vi "Tx Cyclic Init.vi"(8 "error in (no error)":errorcluster, 9 "Channel Number":u32, 10 "signal list":refnum<k21>[](array[refnum])=["CANCyclicSignal1\nnixnet_example.CAN_Cluster", "CANCyclicSignal2\nnixnet_example.CAN_Cluster", "CANCyclicSignal3\nnixnet_example.CAN_Cluster"], 11 "FPGA Refnum":T1) -> (0 "error out":errorcluster, 3 "Tx Cyclic":T2)   [LabVIEW 2020, in "985x Support Addon Engine.lvlib"]
uses:
  985x Support Addon Engine.lvlib
  <resource>/objmgr/xnet.rc
  <vilib>/xnet/xnet.llb/XNET Create Session (Conversion).vi
  Types/Cyclic Frame Info.ctl
  Types/Tx Cyclic Session.ctl
  Types/FPGA Refnum.ctl
  <vilib>/rvi/interface/nirviMethod/nirviMethod.xnode
  <vilib>/FPGAPlugInAG/Dynamic/niLvFpga_ConfigureFifo_Dynamic.vi
  <vilib>/rvi/errors/niLvFpgaMergeErrorWithErrorCode.vi
  <vilib>/FPGAPlugInAG/Dynamic/niLvFpga_StartFifo_Dynamic.vi
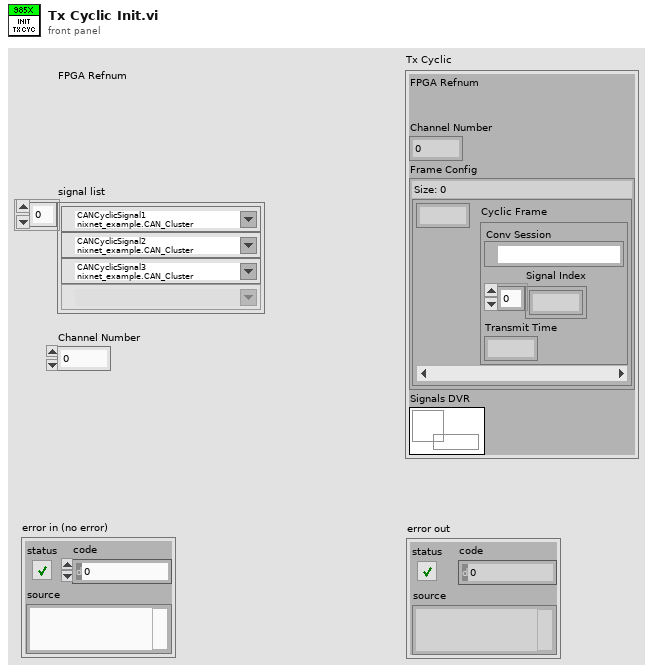
[diagram p1: front panel]
types:
  T1 = typedef "985x Support Addon Engine.lvlib/FPGA Refnum.ctl" = refnum<k20>
  T2 = typedef "985x Support Addon Engine.lvlib/Tx Cyclic Session.ctl" = cluster{"FPGA Refnum":T1, "Channel Number":u32, "Frame Config":map{u32, T3}, "Signals DVR":refnum<data-value>}
  T3 = typedef "985x Support Addon Engine.lvlib/Cyclic Frame Info.ctl" = cluster{"Conv Session":refnum<k21>, "Signal Index":u32[], "Transmit Time":dbl}
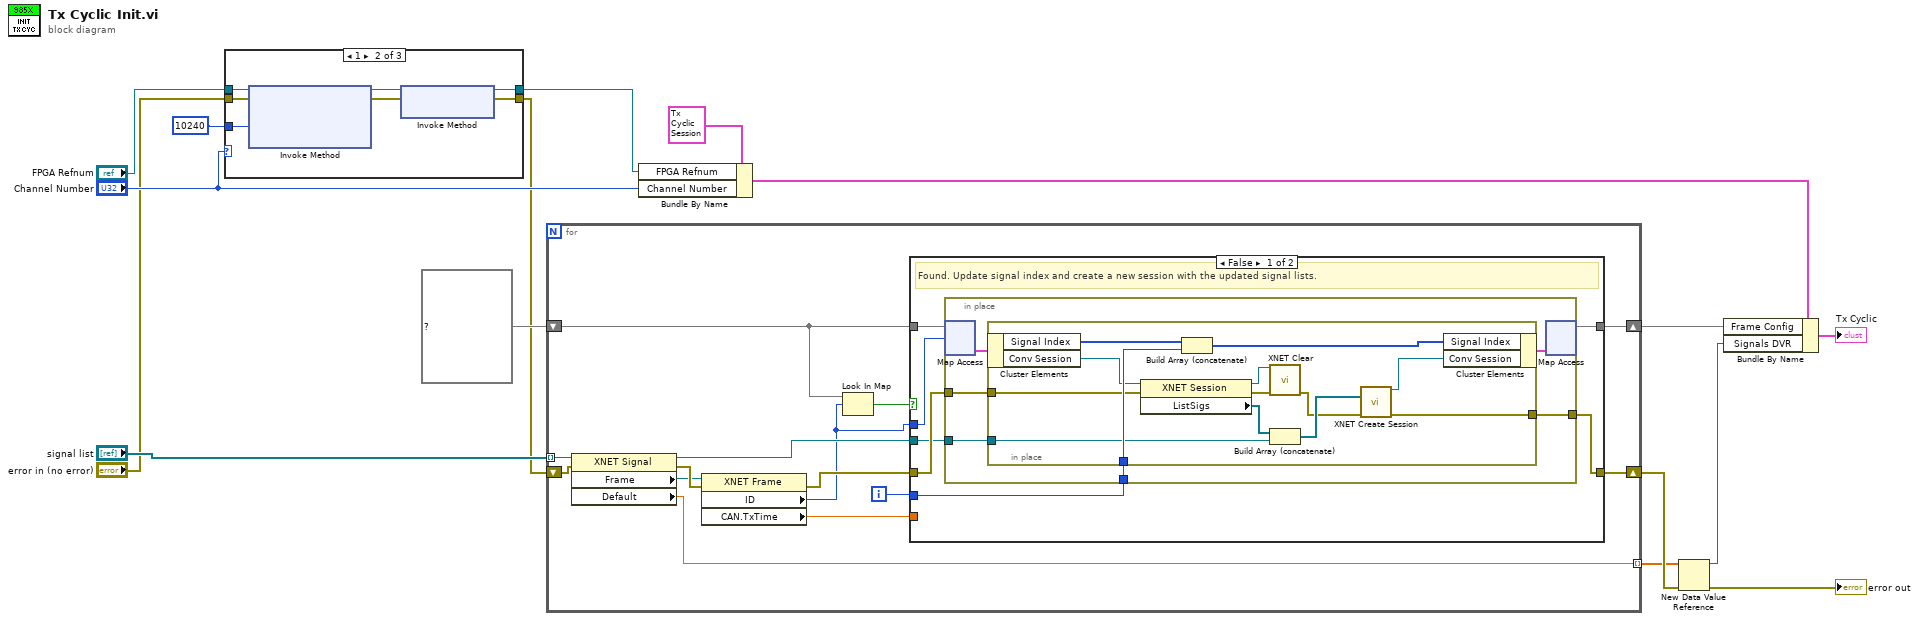
[diagram p0: block diagram]
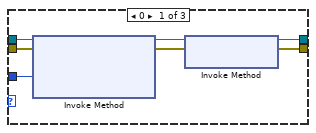
[diagram p2: hidden frame]
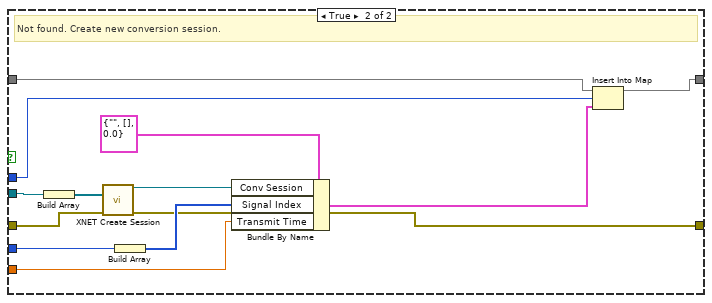
[diagram p4: hidden frame]
diagram:
  n1 = case shown="1" "Channel Number" {
    tunnel: "FPGA Refnum" -> [w23 w30 w32]
    tunnel: "error in (no error)" -> [w22 w29 w31]
    tunnel: u32 10240 ("Requested Depth") -> [w19 w26 _]
    tunnel: [w18 w25 w32] -> w1
    tunnel: [w17 w24 w31] -> w2
    frame 0 {
      n2 = xnode "Invoke Method"("FPGA VI Reference In"=w23, "error in"=w22, "Requested Depth"=w19) -> ("FPGA VI Reference Out"=w21:T1, "error out"=w20:errorcluster)  [unwired: 1 out]
      n3 = xnode "Invoke Method"("FPGA VI Reference In"=w21, "error in"=w20) -> ("FPGA VI Reference Out"=w18:T1, "error out"=w17:errorcluster)
    }
    frame 1 {
      n4 = xnode "Invoke Method"("FPGA VI Reference In"=w30, "error in"=w29, "Requested Depth"=w26) -> ("FPGA VI Reference Out"=w28:T1, "error out"=w27:errorcluster)  [unwired: 1 out]
      n5 = xnode "Invoke Method"("FPGA VI Reference In"=w28, "error in"=w27) -> ("FPGA VI Reference Out"=w25:T1, "error out"=w24:errorcluster)
    }
    frame Default {
    }
  }
  n6 = for {
    tunnel: "signal list" -> [w44] mode=indexing
    shift-right: [w36] -> w11
    shift-left: map{u32, T3} {} ("Frame Config") -> [w41]
    tunnel: [w34] -> w9 mode=indexing
    shift-right: [w33] -> w10
    shift-left: w2 -> [w37]
    i -> [w39]
    n7 = property class="XNET Signal"(reference=w44, error in=w37) -> (reference out=w43:refnum<k21>, error out=w46:errorcluster, "Frame"=w45:refnum<k21>, "Default"=w34:dbl)
    n8 = property class="XNET Frame"(reference=w45, error in=w46) -> (error out=w42:errorcluster, "ID"=w38:u32, "CAN.TxTime"=w35:dbl)  [unwired: 1 out]
    n9 = Look In Map(map=w41, key=w38) -> (key not found?=w40:bool)  [unwired: 1 in, 1 out]
    n10 = case shown="False" w40 {
      tunnel: w41 -> [w53 w85]
      tunnel: w38 -> [w52 w84]
      tunnel: w43 -> [w48 w83]
      tunnel: w42 -> [w49 w81]
      tunnel: w39 -> [w51 w79]
      tunnel: [w47 w76] -> w33
      tunnel: [w50 w75] -> w36
      tunnel: w35 -> [_ w73]
      frame False {
        # "Found. Update signal index and create a new session with the updated signal lists."
        n11 = in-place {
          in-place-border: w51 -> [w58]
          in-place-border: w49 -> [w56]
          in-place-border: w48 -> [w55]
          in-place-border: [w54] -> w47
          n12 = in-place-map #1(w53, w52) -> (w59:T3)  [unwired: 1 in, 1 out]
          n13 = in-place {
            in-place-border: w58 -> [w71]
            in-place-border: w56 -> [w67]
            in-place-border: w55 -> [w66]
            in-place-border: [w60] -> w54
            n14 = in-place-cluster #2(w59) -> ("Signal Index"=w72:u32[], "Conv Session"=w69:refnum<k21>)
            n15 = property class="XNET Session"(reference=w69, error in=w67) -> (reference out=w64:refnum<k21>, error out=w63:errorcluster, "ListSigs"=w68:refnum<k21>[])
            n16 = Build Array (concatenate)(w72, w71) -> (w70:u32[])
            n17 = call <vilib>:"XNET Clear.vi"("session in"=w64, "error in (no error)"=w63) -> ("error out"=w62:errorcluster)  [unwired: 13 in]
            n18 = Build Array (concatenate)(w68, w66) -> (w65:refnum<k21>[])
            n19 = call-poly <vilib>:"XNET Create Session.vi"("signal list"=w65, "error in (no error)"=w62) -> ("session out"=w61:refnum<k21>, "error out"=w60:errorcluster)  [unwired: 12 in]
            n20 = in-place-cluster #2("Signal Index"=w70, "Conv Session"=w61) -> (w57:T3)
          }
          n21 = in-place-map #1(w57) -> (w50:map{u32, T3})  [unwired: 1 in, 2 out]
        }
      }
      frame True {
        # "Not found. Create new conversion session."
        n22 = Build Array(w83) -> (w82:refnum<k21>[])
        n23 = call-poly <vilib>:"XNET Create Session.vi"("signal list"=w82, "error in (no error)"=w81) -> ("session out"=w80:refnum<k21>, "error out"=w76:errorcluster)  [unwired: 12 in]
        n24 = Build Array(w79) -> (w78:i32[])
        n25 = Bundle By Name(cluster=T3 {"Conv Session"="", "Signal Index"=[], "Transmit Time"=0.0} ("Cyclic Frame Info"), "Conv Session"=w80, "Signal Index"=w78, "Transmit Time"=w73) -> (w77:T3)
        n26 = Insert Into Map(map in=w85, key=w84, value=w77) -> (map out=w75:map{u32, T3})  [unwired: 2 out]
      }
    }
  }
  n27 = Bundle By Name(cluster=T2 {"FPGA Refnum"=refnum, "Channel Number"=0, "Frame Config"={}, "Signals DVR"=refnum} ("Tx Cyclic"), "FPGA Refnum"=w1, "Channel Number"="Channel Number") -> (w12:T2)
  n28 = New Data Value Reference(data value=w9, error in=w10) -> (data value reference=w8:refnum<data-value>, error out=→"error out":errorcluster)
  n29 = Bundle By Name(cluster=w12, "Frame Config"=w11, "Signals DVR"=w8) -> (→"Tx Cyclic":T2)
